vi "Addressing.vi"(8 "error in (no error)":errorcluster, 11 "Toolbox in":refnum<class "Toolbox.lvclass">) -> (0 "error out":errorcluster, 2 "Devices_Addresed":i32, 3 "Toolbox out":refnum<class "Toolbox.lvclass">)   [LabVIEW 2014, in "Driver_interaction.lvlib" / "Toolbox.lvclass"]
uses:
  Toolbox.lvclass
  _Driver_interaction/_Driver_interaction.lvclass
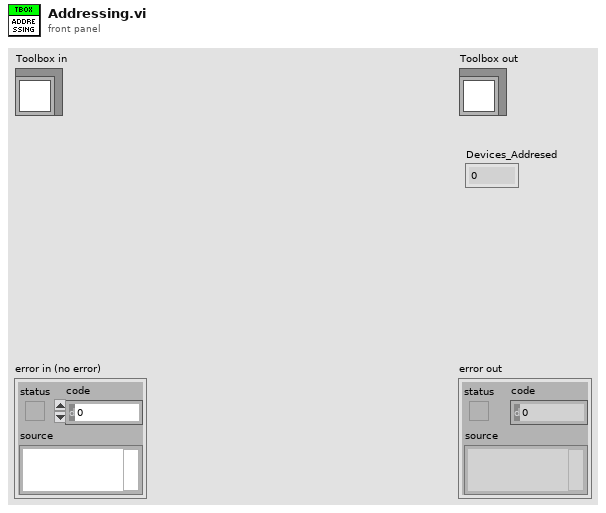
[diagram p1: front panel]
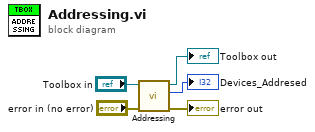
[diagram p0: block diagram]
diagram:
  n1 = call-parent "Addressing.vi"("error in (no error)"="error in (no error)", "_Driver_interaction in"="Toolbox in") -> ("error out"=→"error out":errorcluster, "Devices_Addresed"=→"Devices_Addresed":i32, "_Driver_interaction out"=→"Toolbox out":refnum<class "Toolbox.lvclass">)  [unwired: 7 in]
